vi "飞.vi"(8 "error in (no error)":errorcluster caption="错误输入（无错误）", 11 "橡皮鸭 输入":refnum<class "橡皮鸭.lvclass">) -> (0 "error out":errorcluster caption="错误输出", 3 "橡皮鸭 输出":refnum<class "橡皮鸭.lvclass">)   [LabVIEW 2022 SP3, in "鸭子库.lvlib" / "橡皮鸭.lvclass"]
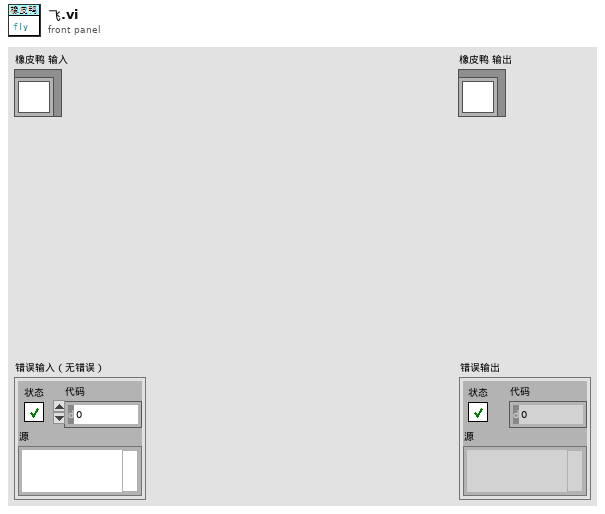
[diagram p1: front panel]
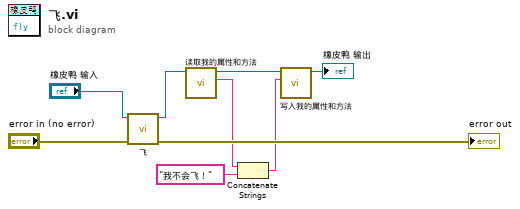
[diagram p0: block diagram]
diagram:
  n1 = call-parent "飞.vi"("error in (no error)"="error in (no error)", "鸭子 输入"="橡皮鸭 输入") -> ("error out"=→"error out":errorcluster, "鸭子 输出"=w5:refnum<class "橡皮鸭.lvclass">)  [unwired: 8 in]
  n2 = call "读取我的属性和方法.vi"("鸭子输入"=w5) -> ("我的属性和方法"=w4:string, "鸭子输出"=w1:refnum<class "橡皮鸭.lvclass">)  [unwired: 8 in, 1 out]
  n3 = Concatenate Strings(w4, "我不会飞！" ("字符串")) -> (w2:string)
  n4 = call "写入我的属性和方法.vi"("我的属性和方法"=w2, "鸭子输入"=w1) -> ("鸭子输出"=→"橡皮鸭 输出":refnum<class "橡皮鸭.lvclass">)  [unwired: 8 in, 1 out]
